vi "Periodic Tasks.vi"   [LabVIEW 2016]
doc: "This VI runs in parallel to other tasks. It can contain as many user-defined periodic loops as you need. These can carry out PID or other sorts of timed response."
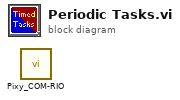
[diagram p0: block diagram]
diagram:
  n1 = call "Pixy_COM-RIO.vi"() -> ()  [unwired: 12 in]
